vi "Test_Config.vi"() -> ()   [LabVIEW 2019]
uses:
  AutoMenuCreator.lvlib
  Ctl/Ctl_Config_Main.ctl
  Ctl/Ctl_Config_File Filter.ctl
  Ctl/Ctl_Config_Folder Filter.ctl
  Ctl/Ctl_Config_Name Edit.ctl
  Ctl/Ctl_Config_Folder Icon Map.ctl
  Ctl/Ctl_Config.ctl
  <vilib>/Palette API/Palette Menu/Public Type Define/View Format.ctl
  <vilib>/Palette API/Palette Menu/Palette Menu.lvlib
  Ctl/Ctl_Config_Palette Data.ctl
  Ctl/Ctl_Config_File Data.ctl
panel:
  out "error out":errorcluster
  out "Config":T1={"Main"={"Menu Folder"="", "Re-Create Menu Folder?"=FALSE, "Allow mnu replace?"=FALSE}, "File Filter"={"Exclude Prefixes"=[], "Ignore Names"=[], "Include Extensions"=[], "Exclude Postfixes"=[]}, "Folder Filter"={"Exclude Prefixes"=[], "Ignore Names"=[]}, "File Name Edit"={"Pre Split String"="", "Post Split String"="", "Deletion Strings"=[]}, "Folder Name Edit"={"Pre Split String"="", "Post Split String"="", "Deletion Strings"=[]}, "Folder Icon Map"={}, "Default Palette Data"={"Display Name Override"="", "View Format"=2, "Palette Width"=0, "Help Tag"="", "Help File Path"=path "", "Palette Description"=""}, "Default File Data"={"Display Name Override"="", "Place VI Contents?"=FALSE}, "Palette Override map"={}, "File Override map"={}} {"Default Palette Data"."View Format" items=["Icons", "Text", "Icons and Text"]}
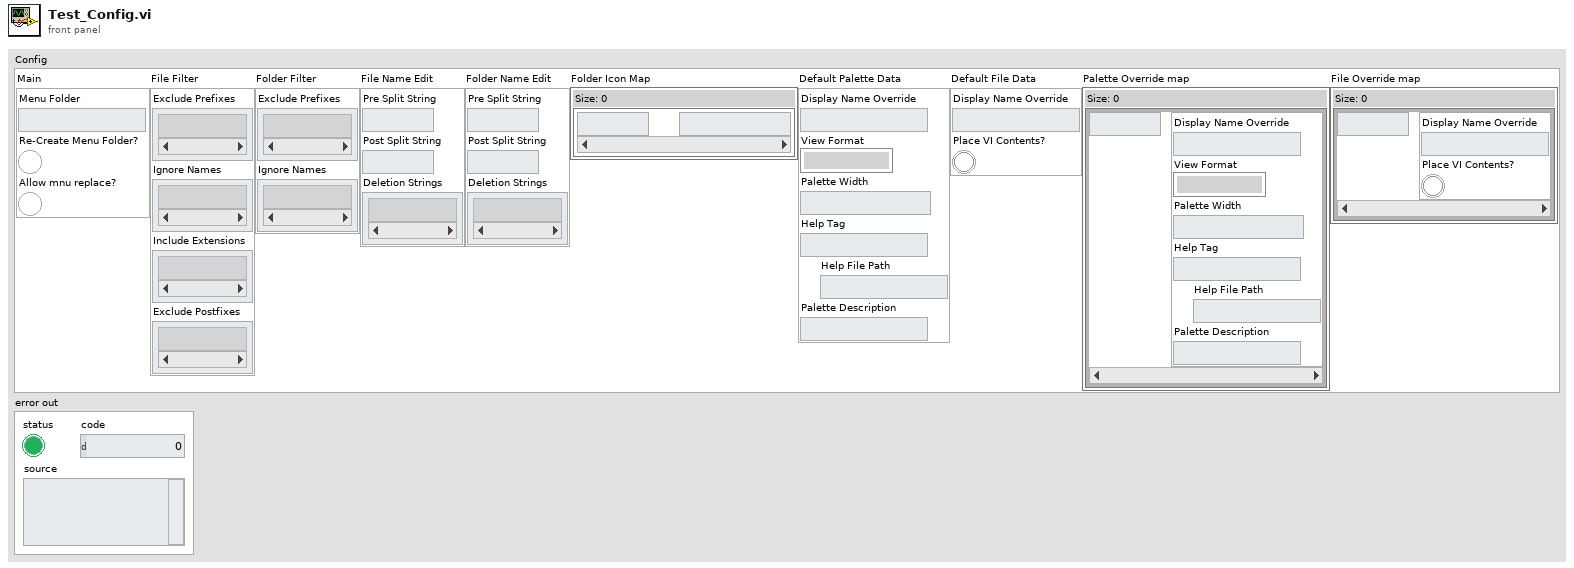
[diagram p1: front panel]
types:
  T1 = typedef "AutoMenuCreator.lvlib/Ctl_Config.ctl" = cluster{"Main":T2, "File Filter":T3, "Folder Filter":T4, "File Name Edit":T5, "Folder Name Edit":T5, "Folder Icon Map":T6, "Default Palette Data":T7, "Default File Data":T9, "Palette Override map":map{string, T7}, "File Override map":map{string, T9}}
  T2 = typedef "AutoMenuCreator.lvlib/Ctl_Config_Main.ctl" = cluster{"Menu Folder":string, "Re-Create Menu Folder?":bool, "Allow mnu replace?":bool}
  T3 = typedef "AutoMenuCreator.lvlib/Ctl_Config_File Filter.ctl" = cluster{"Exclude Prefixes":string[], "Ignore Names":string[], "Include Extensions":string[], "Exclude Postfixes":string[]}
  T4 = typedef "AutoMenuCreator.lvlib/Ctl_Config_Folder Filter.ctl" = cluster{"Exclude Prefixes":string[], "Ignore Names":string[]}
  T5 = typedef "AutoMenuCreator.lvlib/Ctl_Config_Name Edit.ctl" = cluster{"Pre Split String":string, "Post Split String":string, "Deletion Strings":string[]}
  T6 = typedef "AutoMenuCreator.lvlib/Ctl_Config_Folder Icon Map.ctl" = map{string, path}
  T7 = typedef "AutoMenuCreator.lvlib/Ctl_Config_Palette Data.ctl" = cluster{"Display Name Override":string, "View Format":T8, "Palette Width":i16, "Help Tag":string, "Help File Path":path, "Palette Description":string}
  T8 = typedef "Palette Menu.lvlib/View Format.ctl" = u16
  T9 = typedef "AutoMenuCreator.lvlib/Ctl_Config_File Data.ctl" = cluster{"Display Name Override":string, "Place VI Contents?":bool}
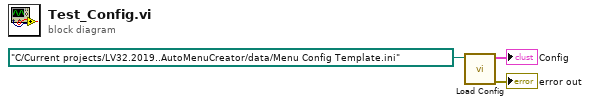
[diagram p0: block diagram]
diagram:
  n1 = call "Load Config.vi"("Target Folder"=path "C:/Current projects/LV32.2019..AutoMenuCreator/data/Menu Config Template.ini") -> ("error out"=→"error out":errorcluster, "Config"=→"Config":T1)  [unwired: 9 in]
